vi "DSF.Shared.Configuration.Transfer.Set Byte Order.vi"(10 "byte order":T1, 11 "Transfer Configuration in":refnum<class "DSF.Shared.Configuration.Transfer.lvclass">) -> (3 "Transfer Configuration out":refnum<class "DSF.Shared.Configuration.Transfer.lvclass">)   [LabVIEW 2017, in "DSF.Engine.lvlib" / "DSF.Shared.Configuration.Transfer.lvclass"]
uses:
  DSF.Shared.Configuration.Transfer.lvclass
  DSF Configuration API/1.0.0/Public/Controls/DSF Byte Order.ctl
  DSF.Shared.Configuration.Transfer.lvclass/DSF.Shared.Configuration.Transfer.ctl
  DSF Configuration API/1.0.0/DSF Configuration API.lvlib
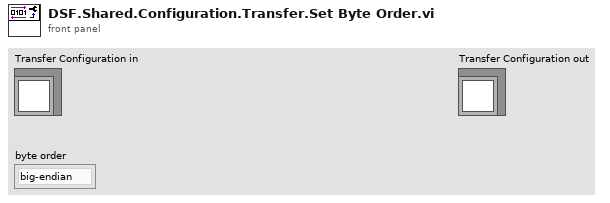
[diagram p1: front panel]
types:
  T1 = typedef "DSF Configuration API.lvlib/DSF Byte Order.ctl" = enum8{"big-endian", "little-endian"}
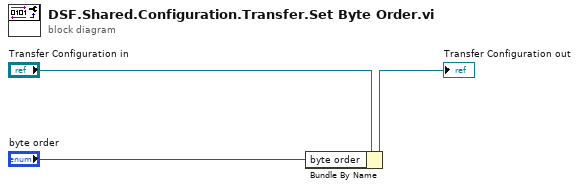
[diagram p0: block diagram]
diagram:
  n1 = Bundle By Name(cluster="Transfer Configuration in", "byte order"="byte order") -> (→"Transfer Configuration out":refnum<class "DSF.Shared.Configuration.Transfer.lvclass">)
